vi "Enable-Disable DIO Bits To Inhibit Motion.vi"(4 "error in (no error)":errorcluster, 5 "Enable DIO Bits to inhibit motion (disable)":bool, 6 "Axis (1)":i32=1 min=1 max=3, 7 "VISA resource name":refnum<visa-resource-name>) -> (0 "error out":errorcluster, 3 "VISA resource name out":refnum<visa-resource-name>)   [LabVIEW 2018, in "Newport ESP301.lvlib"]
doc: "This command is used to disable or enable motion inhibition of requested axes through DIO bits"
uses:
  Newport ESP301.lvlib
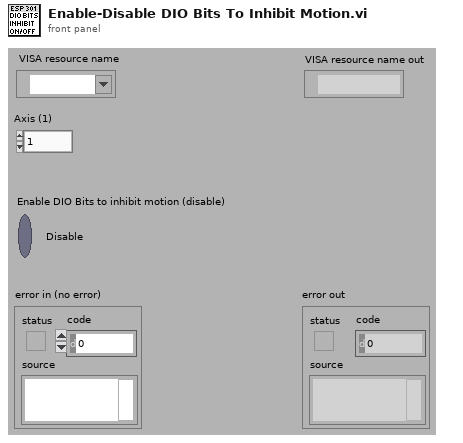
[diagram p1: front panel]
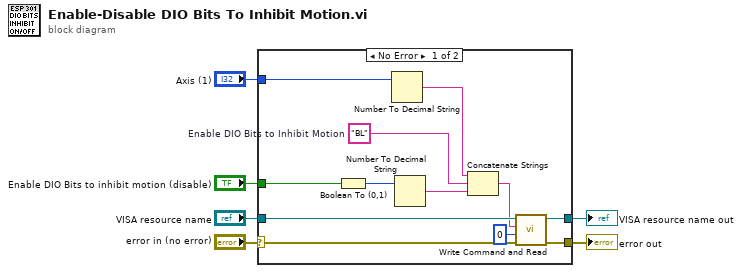
[diagram p0: block diagram]
diagram:
  n1 = case shown="No Error" "error in (no error)" {
    selector: "error in (no error)" -> [w17 w20]
    tunnel: [w16 w20] -> w6
    tunnel: "VISA resource name" -> [w18 w19]
    tunnel: [w15 w19] -> w5
    tunnel: "Axis (1)" -> [w11 _]
    tunnel: "Enable DIO Bits to inhibit motion (disable)" -> [w9 _]
    frame No Error {
      w12 = "BL"  # Enable DIO Bits to Inhibit Motion
      n2 = Boolean To (0,1)(Boolean=w9) -> (0, 1=w13:i16)
      n3 = Number To Decimal String(number=w11) -> (decimal integer string=w14:string)  [unwired: 1 out]
      n4 = Number To Decimal String(number=w13) -> (decimal integer string=w7:string)  [unwired: 1 out]
      n5 = Concatenate Strings(w14, w12, w7) -> (w10:string)
      n6 = call "Write Command and Read.vi"("error in (no error)"=w17, "Bytes to read (100)"=u32 0, "Command"=w10, "VISA resource name"=w18) -> ("error out"=w16:errorcluster, "VISA resource name out"=w15:refnum<visa-resource-name>)  [unwired: 1 in, 3 out]
    }
    frame Error {
    }
  }
  "error out" <- w6
  "VISA resource name out" <- w5
